vi "Read Design Request.vi"(8 "error in":errorcluster) -> (0 "error out":errorcluster, 1 "Number of Pending Requests":i32, 2 "Request Pending":bool, 3 "DesignRequest":T1)   [LabVIEW 2015]
uses:
  Folders.ctl
  user project design.ctl
  Variable cluster.ctl
  Design Request.ctl
panel:
  in  "request datatype":T3
  out "filenames":string[](array[string])
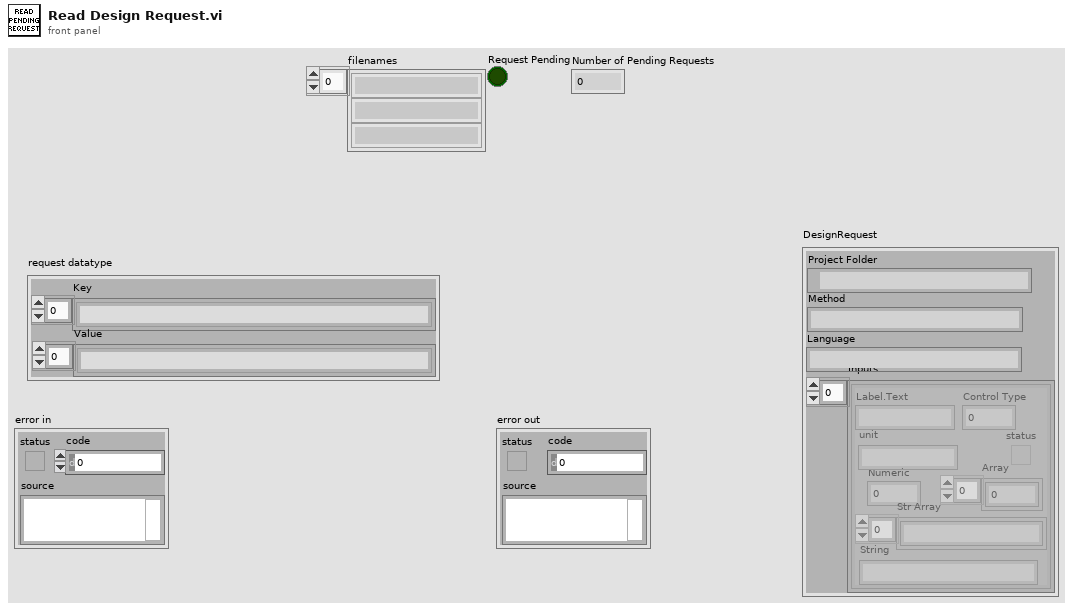
[diagram p1: front panel]
types:
  T1 = typedef "Design Request.ctl" = cluster{"Project Folder":path, "Method":string, "Inputs":T2, "Language":string}
  T2 = typedef "Variable cluster.ctl" = cluster{"Label.Text":string, "Control Type":u32, "Numeric":dbl, "Array":dbl[], "status":bool, "Str Array":string[], "String":string, "unit":string}[]
  T3 = typedef "user project design.ctl" = cluster{"Key":string[], "Value":string[]}
  T4 = typedef "Folders.ctl" = enum16{"DesignTool", "RequestedDesigns", "CompletedDesigns"}
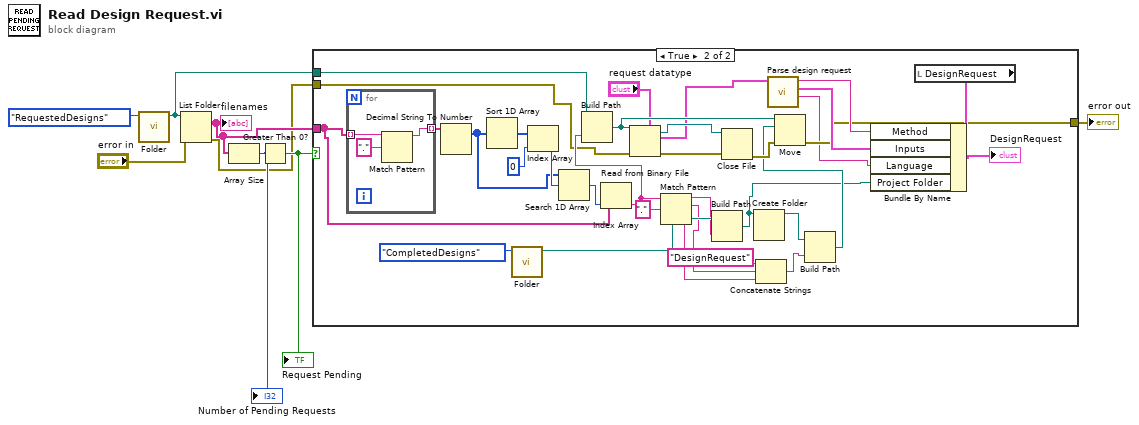
[diagram p0: block diagram]
diagram:
  n1 = call "Folder.vi"("Folders"=Folders."RequestedDesigns") -> ("FolderPath"=w4:path)  [unwired: 9 in, 1 out]
  n2 = List Folder(path=w4, error in="error in") -> (filenames=w7:string[], error out=w2:errorcluster)  [unwired: 2 in, 2 out]
  "filenames" <- w7
  n3 = Array Size(array=w7) -> (size(s)=w6:i32)
  "Number of Pending Requests" <- w6
  n4 = Greater Than 0?(x=w6) -> (x > 0?=w5:bool)
  "Request Pending" <- w5
  n5 = case shown="True" w5 {
    tunnel: w7 -> [_ w36]
    tunnel: w4 -> [_ w40]
    tunnel: w2 -> [w9 w12]
    tunnel: [w9 w11] -> w1
    frame False {
    }
    frame True {
      n6 = for {
        tunnel: w36 -> [w45] mode=indexing
        tunnel: [w43] -> w35 mode=indexing
        n7 = Match Pattern(string=w45, regular expression=".") -> (before substring=w43:string)  [unwired: 1 in, 3 out]
      }
      n8 = Decimal String To Number(string=w35) -> (number=w38:i32[])  [unwired: 2 in, 1 out]
      n9 = Sort 1D Array(array=w38) -> (sorted array=w42:i32[])
      n10 = call "Folder.vi"("Folders"=Folders."CompletedDesigns") -> ("FolderPath"=w32:path)  [unwired: 9 in, 1 out]
      n11 = Index Array(array=w42, index=0) -> (element=w39:i32)
      n12 = Search 1D Array(1D array=w38, element=w39) -> (index of element=w37:i32)  [unwired: 1 in]
      n13 = Index Array(array=w36, index=w37) -> (element=w26:string)
      n14 = Build Path(base path=w40, name or relative path=w26) -> (appended path=w34:path)
      n15 = Read from Binary File(5:"request datatype", 8:w12, 11:w34) -> (0:w28:errorcluster, 2:w27:T3, 3:w29:refnum<file>)  [unwired: 3 in, 1 out]
      n16 = Match Pattern(string=w26, regular expression=".") -> (before substring=w24:string, match substring=w20:string, after substring=w21:string)  [unwired: 1 in, 1 out]
      n17 = Build Path(base path=w32, name or relative path=w24) -> (appended path=w15:path)
      n18 = Close File(refnum=w29, error in=w28) -> (error out=w30:errorcluster)  [unwired: 1 out]
      n19 = Create Folder(path (use dialog)=w15) -> (created path=w23:path)  [unwired: 2 in, 2 out]
      n20 = Concatenate Strings("DesignRequest", w20, w21) -> (w19:string)
      n21 = call "Parse design request.vi"("Request"=w27) -> ("Language"=w10:string, "User and project info"=w14:T2, "Method"=w13:string)  [unwired: 8 in]
      n22 = Build Path(base path=w23, name or relative path=w19) -> (appended path=w18:path)
      n23 = Move(source path=w34, error in=w30, 10:w18) -> (error out=w11:errorcluster)  [unwired: 2 in, 2 out]
      n24 = local read "DesignRequest"() -> (w16:T1)
      n25 = Bundle By Name(cluster=w16, "Method"=w13, "Inputs"=w14, "Language"=w10, "Project Folder"=w15) -> (→"DesignRequest":T1)
    }
  }
  "error out" <- w1
